vi "DelayGeneratorCloseSynchronization.vi"(2 "Synchro":T1, 9 "error in (no error)":errorcluster) -> (6 "error out":errorcluster)   [LabVIEW 2009]
uses:
  Controls/DelayGeneratorSynchro.ctl
  Controls/DelayGeneratorCommand.ctl
  Controls/DelayGeneratorState.ctl
  Controls/DelayTarget.ctl
  Aerotech/Controls/AerotechTarget.ctl
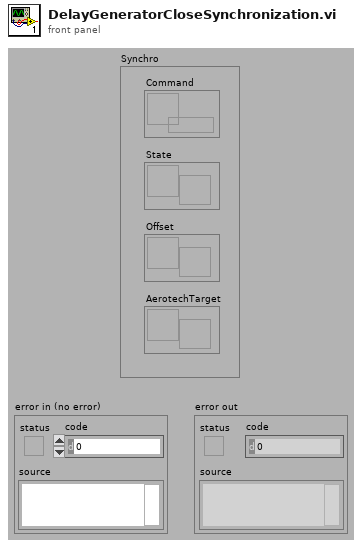
[diagram p1: front panel]
types:
  T1 = typedef "DelayGeneratorSynchro.ctl" = cluster{"Command":refnum<queue>, "State":refnum<notifier>, "Offset":refnum<notifier>, "AerotechTarget":refnum<notifier>}
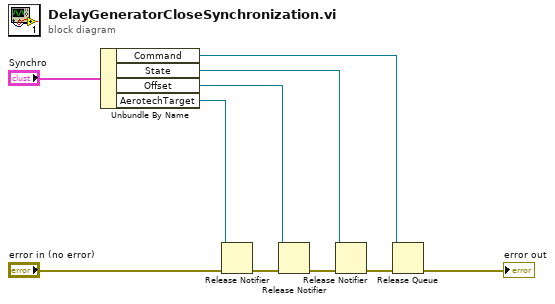
[diagram p0: block diagram]
diagram:
  n1 = Unbundle By Name("Synchro") -> ("Command"=w6:refnum<queue>, "State"=w7:refnum<notifier>, "Offset"=w8:refnum<notifier>, "AerotechTarget"=w9:refnum<notifier>)
  n2 = Release Notifier(notifier=w9, error in (no error)="error in (no error)") -> (error out=w3:errorcluster)  [unwired: 1 in, 2 out]
  n3 = Release Notifier(notifier=w8, error in (no error)=w3) -> (error out=w2:errorcluster)  [unwired: 1 in, 2 out]
  n4 = Release Notifier(notifier=w7, error in (no error)=w2) -> (error out=w1:errorcluster)  [unwired: 1 in, 2 out]
  n5 = Release Queue(queue=w6, error in (no error)=w1) -> (error out=→"error out":errorcluster)  [unwired: 1 in, 2 out]
